vi "DeTurboCode.vi"(0 "appended path":path, 1 "coded_data":dbl[][](array[numeric]), 2 "C":dbl, 3 "Kp":dbl, 4 "error in (no error)":errorcluster caption="错误输入（无错误）") -> (5 "cdblkseg_data":dbl[][](array[numeric]), 6 "error IO":errorcluster)   [LabVIEW 2015]
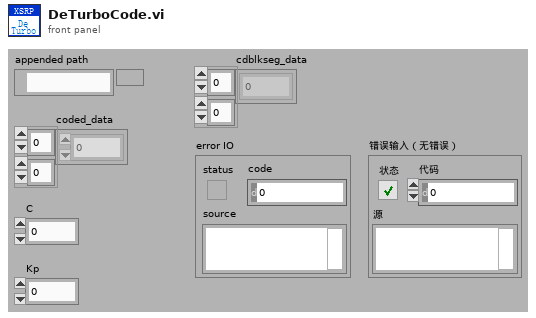
[diagram p1: front panel]
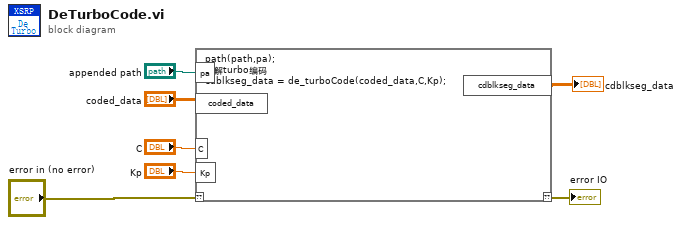
[diagram p0: block diagram]
diagram:
  n1 = script code="path(path,pa);\n%解turbo编码\ncdblkseg_data = de_turboCode(coded_data,C,Kp);"("??"="error in (no error)", "pa"="appended path", "coded_data"="coded_data", "C"="C", "Kp"="Kp") -> ("??"=→"error IO":errorcluster, "cdblkseg_data"=→"cdblkseg_data":dbl[][])
